vi "Launcher.vi"() -> ()   [LabVIEW 2021, in "Recipe.lvlib"]
uses:
  Recipe.lvlib
  Actors/Main Window/Main Window.lvclass
  C:/Program Files (x86)/National Instruments/LabVIEW 2021/vi.lib/MGI/Panel Manager/Panel Actor/Panel Actor/Panel Actor.lvclass
  <vilib>/MGI/Panel Manager/Panel/Window Position/Reference Position/Alignment.ctl
  <vilib>/MGI/Panel Manager/Panel/Window Position/Reference Position/Horizontal Alignment.ctl
  <vilib>/MGI/Panel Manager/Panel/Window Position/Reference Position/Vertical Alignment.ctl
  <vilib>/MGI/Panel Manager/Panel/Window Position/Reference Position/Ref Display/Ref Display.lvclass
  C:/Program Files (x86)/National Instruments/LabVIEW 2021/vi.lib/MGI/Panel Manager/Panel/Window Position/Window Position.lvclass
  <vilib>/MGI/Panel Manager/Panel/Window Position/Reference Position/Ref Display/Ref Display.vi
  <vilib>/MGI/Panel Manager/Panel Actor/Panel Actor/Launch Root Panel Window.vi
  <vilib>/MGI/Panel Manager/Panel Actor/Panel Actor/Panel Actor.lvclass
  <vilib>/MGI/Panel Manager/Panel/Panel.lvlib
  <vilib>/MGI/Monitored Actor/Monitored Actor.lvlib
  <vilib>/MGI/Panel Manager/Panel/Window Position/Reference Position/Reference Position.lvclass
  C:/Program Files (x86)/National Instruments/LabVIEW 2021/vi.lib/MGI/Panel Manager/Panel/Window Position/Reference Position/Reference Position.lvclass
  C:/Program Files (x86)/National Instruments/LabVIEW 2021/vi.lib/MGI/Panel Manager/Panel/Window Position/Reference Position/Ref Display/Ref Display.lvclass
  C:/Program Files (x86)/National Instruments/LabVIEW 2021/vi.lib/MGI/Monitored Actor/Monitored Actor/Monitored Actor/Monitored Actor.lvclass
  C:/Program Files (x86)/National Instruments/LabVIEW 2021/vi.lib/ActorFramework/Actor/Actor.lvclass
  C:/Users/Thomas/Documents/Projects/Recipe/Actors/Main Window/Main Window.lvclass
panel:
  in  "Monitoring?":bool
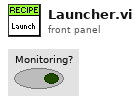
[diagram p1: front panel]
types:
  T1 = typedef "Panel.lvlib/Reference Position.lvclass/Alignment.ctl" = cluster{"Horizontal":T2, "Vertical":T3}
  T2 = typedef "Panel.lvlib/Reference Position.lvclass/Horizontal Alignment.ctl" = enum16{"Left", "Center", "Right"}
  T3 = typedef "Panel.lvlib/Reference Position.lvclass/Vertical Alignment.ctl" = enum16{"Top", "Center", "Bottom"}
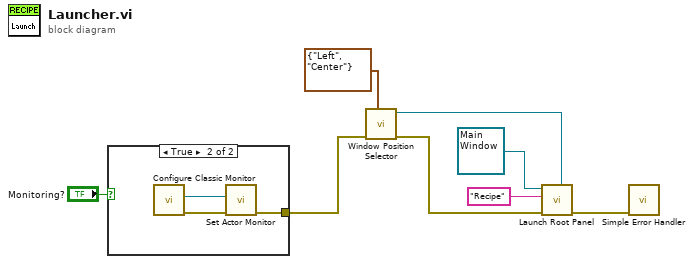
[diagram p0: block diagram]
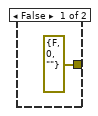
[diagram p2: hidden frame]
diagram:
  n1 = case shown="True" "Monitoring?" {
    tunnel: [errorcluster {"status"=FALSE, "code"=0, "source"=""} ("error out") w12] -> w4
    frame False {
    }
    frame True {
      n2 = call <vilib>:"Configure Classic Monitor.vi"() -> ("error out"=w10:errorcluster, "Classic Monitor out"=w11:refnum<class "Actor Monitor.lvclass">)  [unwired: 10 in]
      n3 = call <vilib>:"Set Actor Monitor.vi"("error in (no error)"=w10, "Actor Monitor"=w11) -> ("error out"=w12:errorcluster)  [unwired: 9 in]
    }
  }
  n4 = call-poly <vilib>:"Window Position Selector.vi"("Alignment"=T1 {"Horizontal"=enum."Left", "Vertical"=enum."Center"}, "Error In"=w4) -> ("Error Out"=w3:errorcluster, "Ref Display out"=w6:refnum<class "Ref Display.lvclass">)  [unwired: 8 in]
  n5 = call-poly <vilib>:"Launch Root Panel.vi"("Window Position (Maximize First Call)"=w6, "Error In"=w3, "Title"="Recipe", "Panel Actor in"=refnum<class "Main Window.lvclass"> refnum ("Recipe.lvlib:Main Window.lvclass")) -> ("Error Out"=w5:errorcluster)  [unwired: 6 in, 1 out]
  n6 = call <vilib>:"Simple Error Handler.vi"("error in (no error)"=w5) -> ()  [unwired: 4 in, 5 out]
